vi "Main.vi"() -> ()   [LabVIEW 2018] (continued)
            n1262 = call <vilib>:"Boolean Crossing PtByPt.vi"("direction"=enum16{"either", "false-true", "true-false"}."false-true", "input"=w6697) -> ("crossing"=w6701:bool)  [unwired: 1 in]
            n1263 = call <vilib>:"Boolean Crossing PtByPt.vi"("direction"=enum16{"either", "false-true", "true-false"}."true-false", "input"=w6697) -> ("crossing"=w6702:bool)  [unwired: 1 in]
            n1264 = call "已用时间6"("Reset"=w6695) -> ("Time has Elapsed"=w6696:bool)  [unwired: 11 in, 7 out]
            n1265 = Insert Into Array(array=bool[] [] ("数组"), index=0 ("索引"), new element #1=w6701, new element #2=w6702) -> (w6705:bool[])
            n1266 = Boolean Array To Number(Boolean array=w6705) -> (number=w6706:u32)
            n1267 = case shown="0, 默认" w6706 {
              tunnel: [cluster{"Data":string[], "State":T1} {"Data"=[], "State"=enum."读扫码请求2"} ("元素") w6725 w6729] -> w6698
              tunnel: w6690 -> [_ w6726 w6730]
              frame 0, Default {
              }
              frame 1 {
                w6725 = cluster{"Data":string[], "State":T1} {"Data"=[], "State"=enum."读数据"} ("元素")
                n1268 = Enqueue Element(queue=w6726, element=w6725, timeout in ms (-1)=10 ("超时毫秒(-1)")) -> ()  [unwired: 1 in, 3 out]
              }
              frame 2 {
                w6729 = cluster{"Data":string[], "State":T1} {"Data"=["999"], "State"=enum."数据保存回复"} ("元素")
                n1269 = Enqueue Element(queue=w6730, element=w6729, timeout in ms (-1)=10 ("超时毫秒(-1)")) -> ()  [unwired: 1 in, 3 out]
              }
            }
            n1270 = case shown="真" w6696 {
              tunnel: w6690 -> [_ w6722]
              frame False {
              }
              frame True {
                n1271 = Enqueue Element(queue=w6722, element=cluster{"Data":string[], "State":T1} {"Data"=["999"], "State"=enum."数据保存回复"} ("元素"), timeout in ms (-1)=10 ("超时毫秒(-1)")) -> ()  [unwired: 1 in, 3 out]
              }
            }
          }
          frame "读数据" {
            w6756 = u16 1 items=["byte", "word", "Dword"] ("数据类型")
            w6760 = u8 132 items=["I/O (P)"=128, "Input (I)"=129, "Output (Q)"=130, "Bit Memory (M)"=131, "Data (DB)"=132, "Instance Data (DI)"=133, "Local Data (L)"=134, "Predecessor Local Data (VL)"=135] ("寄存器类型")
            n1272 = call "S7_Read.vi"("TCP"=w6734, "DB #"=u16 20, "读取长度"=u16 1, "寄存器类型"=w6760, "起始地址"=u32 6, "数据类型"=w6756) -> ("TCP"=w6755:refnum<k5>, "数据"=w6752:u32[], "error out"=w6745:errorcluster)  [unwired: 6 in, 1 out]
            n1273 = local read "ST202 Dowel Pin M0104893"() -> (w6731:string)
            n1274 = Index Array(array=w6752) -> (element=w6751:u32)  [unwired: 1 in]
            n1275 = local read "ST202 Camring 5026187"() -> (w6732:string)
            n1276 = local read "ST202 Rotor 5025805"() -> (w6733:string)
            n1277 = Equal?(x=w6751, y=u32 1) -> (x = y?=w6749:bool)
            n1278 = case shown="假" w6749 {
              tunnel: ["NG" "OK"] -> w6737
              frame False {
              }
              frame True {
              }
            }
            n1279 = Format Date/Time String(time format string (%c)="%Y-%m-%d" ("时间格式字符串(%c)")) -> (date/time string=w6739:string)  [unwired: 2 in]
            n1280 = Get Date/Time String() -> (time string=w6738:string)  [unwired: 3 in, 1 out]
            n1281 = Insert Into Array(array=string[] [] ("数组"), index=0 ("索引"), new element #1="202" ("新元素/子数组"), new element #2=w6737, new element #3=w6739, new element #4=w6738, new element #5=w6737, new element #6=w6733, new element #7=w6732, new element #8=w6731) -> (w6747:string[])
            n1282 = Enqueue Element(queue=w6746, element=w6747, error in (no error)=w6745) -> (error out=w6744:errorcluster)  [unwired: 1 in, 2 out]
            n1283 = property on="ST201数据读取(事件)" class="Bool (严格)"(error in=w6744, "Val(Sgnl)"=TRUE ("值(信号)")) -> (error out=w6735:errorcluster)  [unwired: 1 in, 1 out]
          }
          frame "数据保存回复" {
            w6776 = u8 132 items=["I/O (P)"=128, "Input (I)"=129, "Output (Q)"=130, "Bit Memory (M)"=131, "Data (DB)"=132, "Instance Data (DI)"=133, "Local Data (L)"=134, "Predecessor Local Data (VL)"=135] ("寄存器类型")
            w6777 = u16 1 items=["byte", "word", "Dword"] ("数据类型")
            n1284 = Index Array(array=w6766, index=0 ("索引")) -> (element=w6764:string)
            "数据保存请求回复201" <- w6764
            n1285 = Decimal String To Number(string=w6764, default (0L)=u32 0 ("默认(0 I32)")) -> (number=w6772:u32)  [unwired: 1 in, 1 out]
            n1286 = call "S7_Write.vi"("TCP"=w6771, "寄存器类型"=w6776, "DB #"=u16 20, "写入地址"=u32 4, "数据类型"=w6777, "写入数据"=w6772) -> ("TCP"=w6769:refnum<k5>, "error out"=w6770:errorcluster)  [unwired: 7 in, 1 out]
            n1287 = Bundle By Name(cluster=w6765, "数据保存超时1"=w6764) -> (w6763:T11)
          }
          frame "-----------------" {
          }
          frame "读扫码请求2" {
            w6792 = u8 132 items=["I/O (P)"=128, "Input (I)"=129, "Output (Q)"=130, "Bit Memory (M)"=131, "Data (DB)"=132, "Instance Data (DI)"=133, "Local Data (L)"=134, "Predecessor Local Data (VL)"=135] ("寄存器类型")
            w6793 = u16 1 items=["byte", "word", "Dword"] ("数据类型")
            w6804 = u16 0 items=["byte", "word", "Dword"] ("数据类型")
            w6806 = u8 132 items=["I/O (P)"=128, "Input (I)"=129, "Output (Q)"=130, "Bit Memory (M)"=131, "Data (DB)"=132, "Instance Data (DI)"=133, "Local Data (L)"=134, "Predecessor Local Data (VL)"=135] ("寄存器类型")
            n1288 = Unbundle By Name(w6787) -> ("看门狗"=w6795:string)
            n1289 = Decimal String To Number(string=w6795) -> (number=w6796:i32)  [unwired: 2 in, 1 out]
            n1290 = Equal?(x=w6796, y=0) -> (x = y?=w6798:bool)
            n1291 = case shown="假" w6798 {
              tunnel: [0 ("y") 1 ("y")] -> w6789
              frame False {
              }
              frame True {
              }
            }
            n1292 = local write "20"(w6789) -> ()
            n1293 = call "S7_Write.vi"("TCP"=w6788, "寄存器类型"=w6792, "DB #"=u16 20, "写入地址"=u32 22, "数据类型"=w6793, "写入数据"=w6789) -> ("TCP"=w6785:refnum<k5>, "error out"=w6784:errorcluster)  [unwired: 7 in, 1 out]
            n1294 = Number To Decimal String(number=w6789) -> (decimal integer string=w6790:string)  [unwired: 1 in]
            n1295 = Bundle By Name(cluster=w6787, "看门狗"=w6790) -> (w6786:T11)
            n1296 = call "S7_Read.vi"("TCP"=w6785, "DB #"=u16 20, "读取长度"=u16 1, "寄存器类型"=w6806, "起始地址"=u32 0, "数据类型"=w6804, "error in"=w6784) -> ("TCP"=w6803:refnum<k5>, "数据"=w6829:u32[], "读取成功"=w6816:bool, "error out"=w6800:errorcluster)  [unwired: 5 in]
            n1297 = Not(x=w6816) -> (.not. x?=w6817:bool)
            n1298 = Index Array(array=w6829, index=0 ("索引")) -> (element=w6828:u32)
            n1299 = local write "ST20通讯状态"(w6817) -> ()
            n1300 = Number To Boolean Array(number=w6828) -> (Boolean array=w6827:bool[])
            n1301 = Unbundle By Name(w6786) -> ("扫码超时2"=w6818:string)
            n1302 = Index Array(array=w6827, index=2 ("索引")) -> (element=w6822:bool)
            "ST203扫码请求" <- w6822
            n1303 = Not Equal?(x=w6818, y="999") -> (x != y?=w6819:bool)
            n1304 = Not(x=w6819) -> (.not. x?=w6820:bool)
            n1305 = call <vilib>:"Boolean Crossing PtByPt.vi"("direction"=enum16{"either", "false-true", "true-false"}."false-true", "input"=w6822) -> ("crossing"=w6826:bool)  [unwired: 1 in]
            n1306 = call <vilib>:"Boolean Crossing PtByPt.vi"("direction"=enum16{"either", "false-true", "true-false"}."true-false", "input"=w6822) -> ("crossing"=w6825:bool)  [unwired: 1 in]
            n1307 = call "已用时间21"("Reset"=w6820) -> ("Time has Elapsed"=w6821:bool)  [unwired: 11 in, 7 out]
            n1308 = Insert Into Array(array=bool[] [] ("数组"), index=0 ("索引"), new element #1=w6826, new element #2=w6825) -> (w6824:bool[])
            n1309 = Boolean Array To Number(Boolean array=w6824) -> (number=w6823:u32)
            n1310 = case shown="0, 默认" w6823 {
              tunnel: [cluster{"Data":string[], "State":T1} {"Data"=[], "State"=enum."读数据保存请求2"} ("元素") w6837 w6839] -> w6802
              tunnel: w6799 -> [_ w6838 w6840]
              frame 0, Default {
              }
              frame 1 {
                w6837 = cluster{"Data":string[], "State":T1} {"Data"=[], "State"=enum."读二维码2"} ("元素")
                n1311 = Enqueue Element(queue=w6838, element=w6837, timeout in ms (-1)=10 ("超时毫秒(-1)")) -> ()  [unwired: 1 in, 3 out]
              }
              frame 2 {
                w6839 = cluster{"Data":string[], "State":T1} {"Data"=["999"], "State"=enum."扫码回复2"} ("元素")
                n1312 = Enqueue Element(queue=w6840, element=w6839, timeout in ms (-1)=10 ("超时毫秒(-1)")) -> ()  [unwired: 1 in, 3 out]
              }
            }
            n1313 = case shown="真" w6821 {
              tunnel: w6799 -> [_ w6833]
              frame False {
              }
              frame True {
                n1314 = Enqueue Element(queue=w6833, element=cluster{"Data":string[], "State":T1} {"Data"=["999"], "State"=enum."扫码回复2"} ("元素"), timeout in ms (-1)=10 ("超时毫秒(-1)")) -> ()  [unwired: 1 in, 3 out]
              }
            }
          }
          frame "读二维码2" {
            w6853 = u16 0 items=["byte", "word", "Dword"] ("数据类型")
            w6855 = u8 132 items=["I/O (P)"=128, "Input (I)"=129, "Output (Q)"=130, "Bit Memory (M)"=131, "Data (DB)"=132, "Instance Data (DI)"=133, "Local Data (L)"=134, "Predecessor Local Data (VL)"=135] ("寄存器类型")
            n1315 = call "S7_Read.vi"("TCP"=w6852, "DB #"=u16 20, "读取长度"=u16 17, "寄存器类型"=w6855, "起始地址"=u32 42, "数据类型"=w6853) -> ("TCP"=w6850:refnum<k5>, "数据"=w6858:u32[], "error out"=w6860:errorcluster)  [unwired: 6 in, 1 out]
            n1316 = To Unsigned Word Integer(number=w6858) -> (unsigned 16bit integer=w6859:u16[])
            n1317 = call "还原为字符串.vi"("error in (no error)"=w6860, "输入数组"=w6859) -> ("error out"=w6844:errorcluster, "字符串"=w6845:string)  [unwired: 8 in]
            n1318 = Match Pattern(string=w6845, regular expression=" " ("正则表达式")) -> (before substring=w6842:string)  [unwired: 1 in, 3 out]
            n1319 = flat-sequence {
              tunnel: w6844 -> [w6862]
              tunnel: [w6862] -> w6843
              tunnel: w6842 -> [w6861]
              tunnel: [w6864] -> w6849
              tunnel: w6843 -> [w6863]
              frame #0 {
                "202二维码" <- w6861
              }
              frame #1 {
                n1320 = property on="ST203扫码请求（事件）" class="Bool (严格)"(error in=w6863, "Val(Sgnl)"=TRUE ("值(信号)")) -> (error out=w6864:errorcluster)  [unwired: 1 in, 1 out]
              }
            }
          }
          frame "扫码回复2" {
            n1321 = Array Size(array=w6872) -> (size(s)=w6875:i32)
            n1322 = case shown="3, 默认" w6875 {
              tunnel: w6872 -> [w6877 w6911]
              tunnel: w6873 -> [w6878 w6898]
              tunnel: [w6880 w6889] -> w6870
              tunnel: [w6879 w6888] -> w6869
              tunnel: [w6876 w6887] -> w6874
              frame 1 {
                w6883 = u8 132 items=["I/O (P)"=128, "Input (I)"=129, "Output (Q)"=130, "Bit Memory (M)"=131, "Data (DB)"=132, "Instance Data (DI)"=133, "Local Data (L)"=134, "Predecessor Local Data (VL)"=135] ("寄存器类型")
                w6882 = u16 1 items=["byte", "word", "Dword"] ("数据类型")
                n1323 = Index Array(array=w6877) -> (element=w6876:string)  [unwired: 1 in]
                n1324 = Decimal String To Number(string=w6876, default (0L)=u32 0 ("默认(0 I32)")) -> (number=w6886:u32)  [unwired: 1 in, 1 out]
                n1325 = call "S7_Write.vi"("TCP"=w6878, "寄存器类型"=w6883, "DB #"=u16 20, "写入地址"=u32 14, "数据类型"=w6882, "写入数据"=w6886) -> ("TCP"=w6880:refnum<k5>, "error out"=w6879:errorcluster)  [unwired: 7 in, 1 out]
              }
              frame 3, Default {
                w6901 = u8 132 items=["I/O (P)"=128, "Input (I)"=129, "Output (Q)"=130, "Bit Memory (M)"=131, "Data (DB)"=132, "Instance Data (DI)"=133, "Local Data (L)"=134, "Predecessor Local Data (VL)"=135] ("寄存器类型")
                w6900 = u16 1 items=["byte", "word", "Dword"] ("数据类型")
                w6908 = u8 132 items=["I/O (P)"=128, "Input (I)"=129, "Output (Q)"=130, "Bit Memory (M)"=131, "Data (DB)"=132, "Instance Data (DI)"=133, "Local Data (L)"=134, "Predecessor Local Data (VL)"=135] ("寄存器类型")
                w6909 = u16 1 items=["byte", "word", "Dword"] ("数据类型")
                w6915 = u8 132 items=["I/O (P)"=128, "Input (I)"=129, "Output (Q)"=130, "Bit Memory (M)"=131, "Data (DB)"=132, "Instance Data (DI)"=133, "Local Data (L)"=134, "Predecessor Local Data (VL)"=135] ("寄存器类型")
                w6914 = u16 1 items=["byte", "word", "Dword"] ("数据类型")
                n1326 = Index Array(array=w6911) -> (element #1=w6887:string, element #2=w6894:string, element #3=w6893:string)  [unwired: 3 in]
                n1327 = Equal?(x=w6893, y="OK") -> (x = y?=w6891:bool)
                n1328 = Decimal String To Number(string=w6894, default (0L)=u32 0 ("默认(0 I32)")) -> (number=w6895:u32)  [unwired: 1 in, 1 out]
                n1329 = case shown="假" w6891 {
                  tunnel: [u32 2 ("写入数据") u32 1 ("写入数据")] -> w6890
                  frame False {
                  }
                  frame True {
                  }
                }
                n1330 = call "S7_Write.vi"("TCP"=w6898, "寄存器类型"=w6915, "DB #"=u16 20, "写入地址"=u32 18, "数据类型"=w6914, "写入数据"=w6895) -> ("TCP"=w6905:refnum<k5>, "error out"=w6906:errorcluster)  [unwired: 7 in, 1 out]
                n1331 = call "S7_Write.vi"("TCP"=w6905, "寄存器类型"=w6908, "DB #"=u16 20, "写入地址"=u32 20, "数据类型"=w6909, "写入数据"=w6890, "error in"=w6906) -> ("TCP"=w6897:refnum<k5>, "error out"=w6896:errorcluster)  [unwired: 6 in, 1 out]
                n1332 = Decimal String To Number(string=w6887, default (0L)=u32 0 ("默认(0 I32)")) -> (number=w6904:u32)  [unwired: 1 in, 1 out]
                n1333 = call "S7_Write.vi"("TCP"=w6897, "寄存器类型"=w6901, "DB #"=u16 20, "写入地址"=u32 14, "数据类型"=w6900, "写入数据"=w6904, "error in"=w6896) -> ("TCP"=w6889:refnum<k5>, "error out"=w6888:errorcluster)  [unwired: 6 in, 1 out]
              }
            }
            "扫码请求回复202" <- w6874
            n1334 = Bundle By Name(cluster=w6868, "扫码超时2"=w6874) -> (w6867:T11)
          }
          frame "-- --------------" {
          }
          frame "读数据保存请求2" {
            w6931 = u16 0 items=["byte", "word", "Dword"] ("数据类型")
            w6933 = u8 132 items=["I/O (P)"=128, "Input (I)"=129, "Output (Q)"=130, "Bit Memory (M)"=131, "Data (DB)"=132, "Instance Data (DI)"=133, "Local Data (L)"=134, "Predecessor Local Data (VL)"=135] ("寄存器类型")
            n1335 = call "S7_Read.vi"("TCP"=w6929, "DB #"=u16 20, "读取长度"=u16 1, "寄存器类型"=w6933, "起始地址"=u32 0, "数据类型"=w6931) -> ("TCP"=w6927:refnum<k5>, "数据"=w6954:u32[], "error out"=w6925:errorcluster)  [unwired: 6 in, 1 out]
            n1336 = Index Array(array=w6954, index=0 ("索引")) -> (element=w6953:u32)
            n1337 = Number To Boolean Array(number=w6953) -> (Boolean array=w6952:bool[])
            n1338 = Unbundle By Name(w6930) -> ("数据保存超时2"=w6943:string)
            n1339 = Index Array(array=w6952, index=3 ("索引")) -> (element=w6947:bool)
            "ST202数据读取" <- w6947
            n1340 = Not Equal?(x=w6943, y="999") -> (x != y?=w6944:bool)
            n1341 = Not(x=w6944) -> (.not. x?=w6945:bool)
            n1342 = call <vilib>:"Boolean Crossing PtByPt.vi"("direction"=enum16{"either", "false-true", "true-false"}."false-true", "input"=w6947) -> ("crossing"=w6948:bool)  [unwired: 1 in]
            n1343 = call <vilib>:"Boolean Crossing PtByPt.vi"("direction"=enum16{"either", "false-true", "true-false"}."true-false", "input"=w6947) -> ("crossing"=w6949:bool)  [unwired: 1 in]
            n1344 = call "已用时间22"("Reset"=w6945) -> ("Time has Elapsed"=w6946:bool)  [unwired: 11 in, 7 out]
            n1345 = Insert Into Array(array=bool[] [] ("数组"), index=0 ("索引"), new element #1=w6948, new element #2=w6949) -> (w6950:bool[])
            n1346 = Boolean Array To Number(Boolean array=w6950) -> (number=w6951:u32)
            n1347 = case shown="1" w6951 {
              tunnel: [cluster{"Data":string[], "State":T1} {"Data"=[], "State"=enum."看门狗"} ("元素") w6959 w6963] -> w6924
              tunnel: w6928 -> [_ w6960 w6964]
              frame 0, Default {
              }
              frame 1 {
                w6959 = cluster{"Data":string[], "State":T1} {"Data"=[], "State"=enum."读数据2"} ("元素")
                n1348 = Enqueue Element(queue=w6960, element=w6959, timeout in ms (-1)=10 ("超时毫秒(-1)")) -> ()  [unwired: 1 in, 3 out]
              }
              frame 2 {
                w6963 = cluster{"Data":string[], "State":T1} {"Data"=["999"], "State"=enum."数据保存回复2"} ("元素")
                n1349 = Enqueue Element(queue=w6964, element=w6963, timeout in ms (-1)=10 ("超时毫秒(-1)")) -> ()  [unwired: 1 in, 3 out]
              }
            }
            n1350 = case shown="真" w6946 {
              tunnel: w6928 -> [_ w6956]
              frame False {
              }
              frame True {
                n1351 = Enqueue Element(queue=w6956, element=cluster{"Data":string[], "State":T1} {"Data"=["999"], "State"=enum."数据保存回复2"} ("元素"), timeout in ms (-1)=10 ("超时毫秒(-1)")) -> ()  [unwired: 1 in, 3 out]
              }
            }
          }
          frame "读数据2" {
            w6979 = i16 2 ("精度(6)")
            w6991 = u16 1 items=["byte", "word", "Dword"] ("数据类型")
            w6989 = u8 132 items=["I/O (P)"=128, "Input (I)"=129, "Output (Q)"=130, "Bit Memory (M)"=131, "Data (DB)"=132, "Instance Data (DI)"=133, "Local Data (L)"=134, "Predecessor Local Data (VL)"=135] ("寄存器类型")
            w6993 = u16 1 items=["byte", "word", "Dword"] ("数据类型")
            w6995 = u8 132 items=["I/O (P)"=128, "Input (I)"=129, "Output (Q)"=130, "Bit Memory (M)"=131, "Data (DB)"=132, "Instance Data (DI)"=133, "Local Data (L)"=134, "Predecessor Local Data (VL)"=135] ("寄存器类型")
            n1352 = call "S7_Read.vi"("TCP"=w6986, "DB #"=u16 20, "读取长度"=u16 4, "寄存器类型"=w6989, "起始地址"=u32 60, "数据类型"=w6991) -> ("TCP"=w6981:refnum<k5>, "数据"=w6972:u32[], "error out"=w6980:errorcluster)  [unwired: 6 in, 1 out]
            n1353 = Divide(x=w6972, y=u32[] [100, 100, 100, 100]) -> (x/y=w6974:dbl[])
            n1354 = Index Array(array=w6974) -> (element #1=w6975:dbl, element #2=w6976:dbl, element #3=w6977:dbl, element #4=w6978:dbl)  [unwired: 4 in]
            n1355 = Number To Fractional String(number=w6975, precision (6)=w6979) -> (F-format string=w6971:string)  [unwired: 2 in]
            n1356 = Number To Fractional String(number=w6976, precision (6)=w6979) -> (F-format string=w6970:string)  [unwired: 2 in]
            n1357 = Number To Fractional String(number=w6977, precision (6)=w6979) -> (F-format string=w6969:string)  [unwired: 2 in]
            n1358 = Number To Fractional String(number=w6978, precision (6)=w6979) -> (F-format string=w6968:string)  [unwired: 2 in]
            n1359 = call "S7_Read.vi"("TCP"=w6981, "DB #"=u16 20, "读取长度"=u16 1, "寄存器类型"=w6995, "起始地址"=u32 12, "数据类型"=w6993, "error in"=w6980) -> ("TCP"=w6985:refnum<k5>, "数据"=w7008:u32[], "error out"=w6967:errorcluster)  [unwired: 5 in, 1 out]
            n1360 = Index Array(array=w7008) -> (element=w7007:u32)  [unwired: 1 in]
            n1361 = Equal?(x=w7007, y=u32 1) -> (x = y?=w7006:bool)
            n1362 = case shown="假" w7006 {
              tunnel: ["NG" "OK"] -> w7003
              frame False {
              }
              frame True {
              }
            }
            n1363 = Format Date/Time String(time format string (%c)="%Y-%m-%d" ("时间格式字符串(%c)")) -> (date/time string=w7005:string)  [unwired: 2 in]
            n1364 = Get Date/Time String() -> (time string=w7004:string)  [unwired: 3 in, 1 out]
            n1365 = Insert Into Array(array=string[] [] ("数组"), index=0 ("索引"), new element #1="203" ("新元素/子数组"), new element #2=w7003, new element #3=w7005, new element #4=w7004, new element #5=w7003, new element #6=w6971, new element #7=w6970, new element #8=w6969, new element #9=w6968) -> (w6965:string[])
            n1366 = flat-sequence {
              tunnel: w6967 -> [w7010]
              tunnel: [w7010] -> w6966
              tunnel: w6965 -> [w7009]
              tunnel: [w7012] -> w6983
              tunnel: w6966 -> [w7011]
              frame #0 {
                "202读取数据" <- w7009
              }
              frame #1 {
                n1367 = property on="ST203数据读取（事件）" class="Bool (严格)"(error in=w7011, "Val(Sgnl)"=TRUE ("值(信号)")) -> (error out=w7012:errorcluster)  [unwired: 1 in, 1 out]
              }
            }
          }
          frame "数据保存回复2" {
            w7027 = u8 132 items=["I/O (P)"=128, "Input (I)"=129, "Output (Q)"=130, "Bit Memory (M)"=131, "Data (DB)"=132, "Instance Data (DI)"=133, "Local Data (L)"=134, "Predecessor Local Data (VL)"=135] ("寄存器类型")
            w7024 = u16 1 items=["byte", "word", "Dword"] ("数据类型")
            n1368 = Index Array(array=w7018, index=0 ("索引")) -> (element=w7030:string)
            "数据保存请求回复202" <- w7030
            n1369 = Decimal String To Number(string=w7030, default (0L)=u32 0 ("默认(0 I32)")) -> (number=w7031:u32)  [unwired: 1 in, 1 out]
            n1370 = call "S7_Write.vi"("TCP"=w7023, "寄存器类型"=w7027, "DB #"=u16 20, "写入地址"=u32 16, "数据类型"=w7024, "写入数据"=w7031) -> ("TCP"=w7020:refnum<k5>, "error out"=w7019:errorcluster)  [unwired: 7 in, 1 out]
            n1371 = Bundle By Name(cluster=w7022, "数据保存超时2"=w7030) -> (w7021:T11)
          }
          frame "------------" {
          }
          frame "错误" {
            n1372 = Flush Queue(queue=w7039) -> ()  [unwired: 1 in, 3 out]
            n1373 = Flush Queue(queue=w7038) -> ()  [unwired: 1 in, 3 out]
            n1374 = call "S7_Close.vi"("TCP Connection Ref"=w7042) -> ("error out"=w7040:errorcluster)  [unwired: 10 in]
            n1375 = call <vilib>:"Clear Errors.vi"("error in (no error)"=w7040) -> ()  [unwired: 5 in, 2 out]
          }
          frame "退出" {
            n1376 = Release Queue(queue=w7051) -> ()  [unwired: 2 in, 3 out]
            n1377 = Release Queue(queue=w7050) -> ()  [unwired: 2 in, 3 out]
            n1378 = call "S7_Close.vi"("TCP Connection Ref"=w7049) -> ("error out"=w7047:errorcluster)  [unwired: 10 in]
          }
          frame "看门狗" {
            w7064 = "\r" ("正则表达式")
            w7082 = u16 0 items=["byte", "word", "Dword"] ("数据类型")
            w7080 = u8 132 items=["I/O (P)"=128, "Input (I)"=129, "Output (Q)"=130, "Bit Memory (M)"=131, "Data (DB)"=132, "Instance Data (DI)"=133, "Local Data (L)"=134, "Predecessor Local Data (VL)"=135] ("寄存器类型")
            w7092 = u8 132 items=["I/O (P)"=128, "Input (I)"=129, "Output (Q)"=130, "Bit Memory (M)"=131, "Data (DB)"=132, "Instance Data (DI)"=133, "Local Data (L)"=134, "Predecessor Local Data (VL)"=135] ("寄存器类型")
            w7093 = u16 1 items=["byte", "word", "Dword"] ("数据类型")
            n1379 = Unbundle By Name(w7085) -> ("看门狗"=w7095:string)
            n1380 = Decimal String To Number(string=w7095) -> (number=w7096:i32)  [unwired: 2 in, 1 out]
            n1381 = Equal?(x=w7096, y=0) -> (x = y?=w7098:bool)
            n1382 = case shown="假" w7098 {
              tunnel: [0 ("y") 1 ("y")] -> w7086
              frame False {
              }
              frame True {
              }
            }
            "20" <- w7086
            n1383 = call "S7_Write.vi"("TCP"=w7090, "寄存器类型"=w7092, "DB #"=u16 20, "写入地址"=u32 22, "数据类型"=w7093, "写入数据"=w7086) -> ("TCP"=w7072:refnum<k5>, "error out"=w7071:errorcluster)  [unwired: 7 in, 1 out]
            n1384 = Number To Decimal String(number=w7086) -> (decimal integer string=w7087:string)  [unwired: 1 in]
            n1385 = Bundle By Name(cluster=w7085, "看门狗"=w7087) -> (w7084:T11)
            n1386 = call "S7_Read.vi"("TCP"=w7072, "DB #"=u16 20, "读取长度"=u16 120, "寄存器类型"=w7080, "起始地址"=u32 70, "数据类型"=w7082, "error in"=w7071) -> ("TCP"=w7057:refnum<k5>, "数据"=w7074:u32[], "error out"=w7056:errorcluster)  [unwired: 5 in, 1 out]
            n1387 = To Unsigned Word Integer(number=w7074) -> (unsigned 16bit integer=w7073:u16[])
            n1388 = call "还原为字符串.vi"("输入数组"=w7073) -> ("字符串"=w7075:string)  [unwired: 9 in, 1 out]
            n1389 = for {
              N: 6 -> [_]
              tunnel: w7075 -> [w7115]
              tunnel: [w7114] -> w7083 mode=indexing
              shift-right: [w7110] -> _
              shift-left: 0 ("长度（剩余）") -> [w7112]
              n1390 = String Subset(string=w7115, offset (0)=w7112, length (rest)=20 ("长度（剩余）")) -> (substring=w7114:string)
              n1391 = Add(x=w7112, y=20) -> (x+y=w7110:i32)
            }
            n1392 = Index Array(array=w7083) -> (element #1=w7070:string, element #2=w7069:string, element #3=w7068:string, element #4=w7067:string, element #5=w7066:string, element #6=w7065:string)  [unwired: 6 in]
            n1393 = Match Pattern(string=w7070, regular expression=w7064) -> (before substring=→"ST202 Rotor 5025805":string)  [unwired: 1 in, 3 out]
            n1394 = Match Pattern(string=w7069, regular expression=w7064) -> (before substring=→"ST202 Camring 5026187":string)  [unwired: 1 in, 3 out]
            n1395 = Match Pattern(string=w7068, regular expression=w7064) -> (before substring=→"ST202 Dowel Pin M0104893":string)  [unwired: 1 in, 3 out]
            n1396 = Match Pattern(string=w7067, regular expression=w7064) -> (before substring=→"ST301 Vane 5004737":string)  [unwired: 1 in, 3 out]
            n1397 = Match Pattern(string=w7066, regular expression=w7064) -> (before substring=→"ST301 Dowel Pin 5024533":string)  [unwired: 1 in, 3 out]
            n1398 = Match Pattern(string=w7065, regular expression=w7064) -> (before substring=→"ST301 Dowel Pin 5020282":string)  [unwired: 1 in, 3 out]
            n1399 = disable-structure shown="启用" {
              disable-tunnel: w7057 -> [w7099 w7103]
              disable-tunnel: [w7099 w7106] -> w7054
              disable-tunnel: w7056 -> [w7100 w7104]
              disable-tunnel: [w7100 w7105] -> w7055
              frame Disabled {
              }
              frame Enabled {
                w7108 = u8 132 items=["I/O (P)"=128, "Input (I)"=129, "Output (Q)"=130, "Bit Memory (M)"=131, "Data (DB)"=132, "Instance Data (DI)"=133, "Local Data (L)"=134, "Predecessor Local Data (VL)"=135] ("寄存器类型")
                w7102 = u16 1 items=["byte", "word", "Dword"] ("数据类型")
                n1400 = local read "80产品型号"() -> (w7101:u32)
                n1401 = call "S7_Write.vi"("TCP"=w7103, "寄存器类型"=w7108, "DB #"=u16 20, "写入地址"=u32 190, "数据类型"=w7102, "写入数据"=w7101, "error in"=w7104) -> ("TCP"=w7106:refnum<k5>, "error out"=w7105:errorcluster)  [unwired: 6 in, 1 out]
              }
            }
          }
        }
      }
      n1402 = while {
        tunnel: w107 -> [w613]
        tunnel: w144 -> [w612]
        stop <- w611 stop-if-true
        n1403 = event shown="[0] 超时" {
          selector: _ -> [_ _ _ _ _ _ _ _ _ _ _ _]
          dyn-events: _ -> [_ _ _ _ _ _ _ _ _ _ _ _]
          timeout: 10 -> [_ _ _ _ _ _ _ _ _ _ _ _]
          tunnel: w613 -> [_ w621 _ _ _ _ _ _ _ _ _ _]
          tunnel: w612 -> [_ w620 _ _ _ _ _ _ _ _ _ _]
          tunnel: [FALSE w617 FALSE FALSE FALSE FALSE FALSE FALSE FALSE FALSE FALSE FALSE] -> w611
          event Timeout {
            n1404 = event-data() -> ()  [unwired: 1 in, 3 out]
          }
          event Panel Close {
            n1405 = event-data() -> ()  [unwired: 1 in, 3 out]
            n1406 = call <vilib>:"DB Tools Close Connection.vi"("error in (no error)"=w621, "connection reference"=w620) -> ()  [unwired: 5 in, 1 out]
            n1407 = Two Button Dialog(message="确定退出？" ("消息")) -> (T button?=w618:bool)  [unwired: 2 in]
            n1408 = case shown="真" w618 {
              tunnel: [FALSE TRUE] -> w617
              frame False {
              }
              frame True {
                n1409 = flat-sequence {
                  frame #0 {
                    n1410 = property on="错误信息" class="LstBox (严格)"() -> ("Item Names"=w626:string[])  [unwired: 2 in, 2 out]
                    n1411 = Array Size(array=w626) -> (size(s)=w625:i32)
                    n1412 = Equal To 0?(x=w625) -> (x = 0?=w624:bool)
                    n1413 = case shown="假" w624 {
                      tunnel: w626 -> [w627 _]
                      frame False {
                        n1414 = call <vilib>:"Check if File or Folder Exists.vi"("path"=path "D:/Alarm_Log") -> ("error out"=w643:errorcluster, "file or folder exists?"=w644:bool, "dup path"=w642:path)  [unwired: 8 in]
                        n1415 = case shown="真" w644 {
                          tunnel: w643 -> [w659 w660]
                          tunnel: w642 -> [w658 w661]
                          tunnel: [w657 w661] -> w641
                          tunnel: [w656 w660] -> w636
                          frame False {
                            n1416 = Create Folder(path (use dialog)=w658, error in=w659) -> (created path=w657:path, error out=w656:errorcluster)  [unwired: 1 in, 1 out]
                          }
                          frame True {
                          }
                        }
                        n1417 = Format Date/Time String(time format string (%c)="%Y%m%d" ("时间格式字符串(%c)")) -> (date/time string=w639:string)  [unwired: 2 in]
                        n1418 = Concatenate Strings(w639, ".txt" ("字符串")) -> (w637:string)
                        n1419 = Build Path(base path=w641, name or relative path=w637) -> (appended path=w630:path)
                        n1420 = call <vilib>:"Check if File or Folder Exists.vi"("error in (no error)"=w636, "path"=w630) -> ("error out"=w634:errorcluster, "file or folder exists?"=w635:bool, "dup path"=w633:path)  [unwired: 7 in]
                        n1421 = case shown="假" w635 {
                          tunnel: w634 -> [_ w649]
                          tunnel: w633 -> [_ w648]
                          tunnel: [string[] [] ("array of strings") w647] -> w631
                          frame False {
                          }
                          frame True {
                            n1422 = Read from Text File(file (use dialog)=w648, error in=w649) -> (text=w650:string)  [unwired: 2 in, 3 out]
                            n1423 = Search and Replace String(replace all?=TRUE ("替换全部？(F)"), input string=w650, search string="\n" ("搜索字符串"), replace string="\\" ("替换字符串(\"\")")) -> (result string=w654:string)  [unwired: 4 in, 3 out]
                            n1424 = String To Path(string=w654) -> (path=w655:path)
                            n1425 = Path to Array of Strings(0:w655) -> (2:w647:string[])  [unwired: 1 out]
                          }
                        }
                        n1426 = Array Size(array=w627) -> (size(s)=w632:i32)
                        n1427 = Insert Into Array(array=w627, index=w632, new element=w631) -> (w629:string[])
                        n1428 = Write to Text File(file (use dialog)=w630, text=w629) -> (error out=w628:errorcluster)  [unwired: 2 in, 2 out]
                        n1429 = call <vilib>:"Clear Errors.vi"("error in (no error)"=w628) -> ()  [unwired: 5 in, 2 out]
                      }
                      frame True {
                      }
                    }
                  }
                  frame #1 {
                    n1430 = control-ref of="本VI"() -> (w662:refnum<vi>)
                    n1431 = property class="VI"(reference=w662, "FP.State"=T6."Closed" ("前面板窗口:状态")) -> ()  [unwired: 1 in, 2 out]
                  }
                }
              }
            }
            n1432 = local write "退出"(w617) -> ()
          }
          event "返回": Value Change {
            n1433 = event-data() -> ()  [unwired: 1 in, 3 out]
            n1434 = local write "Main Tab"(T2."Running" ("Main Tab")) -> ()
          }
          event "登录界面": Value Change {
            w666 = "" ("输入管理员密码")
            n1435 = event-data() -> ()  [unwired: 1 in, 3 out]
            n1436 = local write "输入管理员密码"(w666) -> ()
            n1437 = local write "登录状态"(w666) -> ()
            n1438 = local write "Main Tab"(T2."Setting" ("Main Tab")) -> ()
          }
          event "登录": Value Change {
            n1439 = event-data() -> ()  [unwired: 1 in, 3 out]
            n1440 = local read "Code"() -> (w675:string)
            n1441 = Equal?(x="输入管理员密码", y="15505240996") -> (x = y?=w669:bool)
            n1442 = Equal?(x="输入管理员密码", y=w675) -> (x = y?=w674:bool)
            n1443 = case shown="真" w669 {
              frame False {
              }
              frame True {
                "Main Tab" <- T2."Monitor" ("Main Tab")
              }
            }
            n1444 = case shown="真" w674 {
              tunnel: ["登录失败！" ("登录状态") "登录成功！" ("登录状态")] -> w673
              frame False {
              }
              frame True {
                w679 = TRUE ("可见")
                n1445 = property on="Rework界面" class="Bool"("Visible"=w679) -> ()  [unwired: 2 in, 2 out]
                n1446 = property on="修改密码" class="Bool"("Visible"=w679) -> ()  [unwired: 2 in, 2 out]
                n1447 = property on="注销" class="Bool"("Visible"=w679) -> ()  [unwired: 2 in, 2 out]
                n1448 = local write "Main Tab"(T2."Running" ("Main Tab")) -> ()
              }
            }
            "登录状态" <- w673
          }
          event "修改密码界面返回", "登录界面返回", "Rework返回": Value Change {
            n1449 = event-data() -> ()  [unwired: 1 in, 3 out]
            n1450 = local write "Main Tab"(T2."Running" ("Main Tab")) -> ()
          }
          event "Rework界面": Value Change {
            w683 = FALSE ("503")
            w686 = "" ("输入需要Rework的一维码：")
            n1451 = event-data() -> ()  [unwired: 1 in, 3 out]
            n1452 = local write "80"(w683) -> ()
            n1453 = local write "101"(w683) -> ()
            n1454 = local write "102"(w683) -> ()
            n1455 = local write "202"(w683) -> ()
            n1456 = local write "203"(w683) -> ()
            n1457 = local write "301"(w683) -> ()
            n1458 = local write "302"(w683) -> ()
            n1459 = local write "401"(w683) -> ()
            n1460 = local write "403"(w683) -> ()
            n1461 = local write "502"(w683) -> ()
            n1462 = local write "503"(w683) -> ()
            n1463 = local write "601"(w683) -> ()
            n1464 = local write "602"(w683) -> ()
            n1465 = local write "70"(w683) -> ()
            n1466 = local write "Rework状态"(w686) -> ()
            n1467 = local write "输入需要Rework的一维码："(w686) -> ()
            n1468 = local write "Main Tab"(T2."Rework" ("Main Tab")) -> ()
          }
          event "102", "202", "301", "401", "502", "503", "601", "70", "101", "203", "302", "403", "602": Value Change {
            w687 = cluster{u32, u32}[] [{1985280, 1985280}, {6618880, 6618880}, {1985280, 1985280}, {6618880, 6618880}] ("颜色[4]")
            n1469 = event-data() -> ()  [unwired: 1 in, 3 out]
            n1470 = property on="101" class="Bool (严格)"("Colors [4]"=w687) -> ()  [unwired: 2 in, 2 out]
            n1471 = property on="102" class="Bool (严格)"("Colors [4]"=w687) -> ()  [unwired: 2 in, 2 out]
            n1472 = property on="202" class="Bool (严格)"("Colors [4]"=w687) -> ()  [unwired: 2 in, 2 out]
            n1473 = property on="203" class="Bool (严格)"("Colors [4]"=w687) -> ()  [unwired: 2 in, 2 out]
            n1474 = property on="301" class="Bool (严格)"("Colors [4]"=w687) -> ()  [unwired: 2 in, 2 out]
            n1475 = property on="302" class="Bool (严格)"("Colors [4]"=w687) -> ()  [unwired: 2 in, 2 out]
            n1476 = property on="401" class="Bool (严格)"("Colors [4]"=w687) -> ()  [unwired: 2 in, 2 out]
            n1477 = property on="403" class="Bool (严格)"("Colors [4]"=w687) -> ()  [unwired: 2 in, 2 out]
            n1478 = property on="502" class="Bool (严格)"("Colors [4]"=w687) -> ()  [unwired: 2 in, 2 out]
            n1479 = property on="503" class="Bool (严格)"("Colors [4]"=w687) -> ()  [unwired: 2 in, 2 out]
            n1480 = property on="601" class="Bool (严格)"("Colors [4]"=w687) -> ()  [unwired: 2 in, 2 out]
            n1481 = property on="602" class="Bool (严格)"("Colors [4]"=w687) -> ()  [unwired: 2 in, 2 out]
            n1482 = property on="70" class="Bool (严格)"("Colors [4]"=w687) -> ()  [unwired: 2 in, 2 out]
          }
          event "注销": Value Change {
            w689 = FALSE ("可见")
            n1483 = event-data() -> ()  [unwired: 1 in, 3 out]
            n1484 = property on="Rework界面" class="Bool"("Visible"=w689) -> ()  [unwired: 2 in, 2 out]
            n1485 = property on="修改密码" class="Bool"("Visible"=w689) -> ()  [unwired: 2 in, 2 out]
            n1486 = property on="注销" class="Bool"("Visible"=w689) -> ()  [unwired: 2 in, 2 out]
          }
          event "修改密码": Value Change {
            w691 = "" ("修改密码状态")
            n1487 = event-data() -> ()  [unwired: 1 in, 3 out]
            n1488 = local write "Main Tab"(T2."Modify" ("Main Tab")) -> ()
            n1489 = local write "修改密码状态"(w691) -> ()
            n1490 = local write "新密码"(w691) -> ()
            n1491 = local write "初始密码"(w691) -> ()
          }
          event "确认修改密码": Value Change {
            n1492 = event-data() -> ()  [unwired: 1 in, 3 out]
            n1493 = local read "Code"() -> (w696:string)
            n1494 = Equal?(x="初始密码", y=w696) -> (x = y?=w695:bool)
            n1495 = case shown="真" w695 {
              tunnel: ["初始密码错误" ("修改密码状态") w701] -> w694
              frame False {
              }
              frame True {
                w703 = "Code" ("subkeyName")
                n1496 = call "Write Registry.vi"("value"=w703, "data"="新密码", "subkeyName"=w703) -> ("error out"=w702:errorcluster)  [unwired: 8 in]
                n1497 = case shown="无错误" w702 {
                  tunnel: ["修改密码成功" ("修改密码状态") "修改密码失败" ("修改密码状态")] -> w701
                  tunnel: "新密码" -> [w704 _]
                  frame No Error {
                    n1498 = local write "Code"(w704) -> ()
                  }
                  frame Error {
                  }
                }
              }
            }
            "修改密码状态" <- w694
          }
          event "OP70画曲线": Value Change {
            # "注：分支0：未收到请求，查找下一个PLC请求\n      分支1：扫码请求，读取码\n      分支2：扫码复位，回复给PLC的也要复位"
            n1499 = event-data() -> ()  [unwired: 1 in, 3 out]
            n1500 = call "检查曲线文件.vi"("Folder Path"=path "D:/op70" ("路径")) -> ("Error Out"=w709:errorcluster, "Exit?"=w711:bool, "曲线文件路径"=w710:path)  [unwired: 7 in, 1 out]
            n1501 = case shown="真" w711 {
              tunnel: w710 -> [_ w726]
              tunnel: w709 -> [w722 w725]
              tunnel: [w722 w724] -> w708
              frame False {
              }
              frame True {
                n1502 = flat-sequence {
                  tunnel: [w730] -> w727
                  tunnel: w726 -> [w729]
                  tunnel: w725 -> [w731]
                  tunnel: [w729] -> w723
                  tunnel: w727 -> [w744]
                  tunnel: [w749] -> w724
                  tunnel: w723 -> [w747]
                  frame #0 {
                    n1503 = call "EXCEL 画曲线.vi"("错误输入（无错误）"=w731, "路径"=w729) -> ("error IO"=w730:errorcluster, "XY图"=→"XY图":cluster{"X":dbl, "Y":dbl}[])  [unwired: 8 in]
                    "曲线文件路径" <- w729
                  }
                  frame #1 {
                    n1504 = local read "70二维码"() -> (w735:string)
                    n1505 = Format Date/Time String(time format string (%c)="%Y%m%d" ("时间格式字符串(%c)")) -> (date/time string=w732:string)  [unwired: 2 in]
                    n1506 = call "图片保存(subaru).vi"("一维码"=w732) -> ("dup path"=w737:path)  [unwired: 9 in, 1 out]
                    n1507 = Build Path(base path=w737, name or relative path=w735) -> (appended path=w750:path)
                    n1508 = call <vilib>:"Check if File or Folder Exists.vi"("path"=w750) -> ("error out"=w751:errorcluster, "file or folder exists?"=w752:bool)  [unwired: 8 in, 1 out]
                    n1509 = Concatenate Strings(w735, "ST70.BMP" ("字符串")) -> (w753:string)
                    n1510 = case shown="假" w752 {
                      tunnel: w750 -> [w757 w759]
                      tunnel: [w756 w759] -> w736
                      tunnel: w751 -> [w755 w758]
                      tunnel: [w754 w758] -> _
                      frame False {
                        n1511 = Create Folder(path (use dialog)=w757, error in=w755) -> (created path=w756:path, error out=w754:errorcluster)  [unwired: 1 in, 1 out]
                      }
                      frame True {
                      }
                    }
                    n1512 = Build Path(base path=w736, name or relative path=w753) -> (appended path=w746:path)
                    n1513 = call "文件路径.vi"("文件路径"=w746, "文件格式"=".BMP") -> ("新路径"=w740:path)  [unwired: 9 in]
                    n1514 = invoke on="XY图" class="XYGraph (严格)" method="Export Image"(error in=w744, "FileType"=enum32{"BMP", "EPS", "EMF", "PICT"}."BMP" ("文件类型"), "Target"=enum32{"File", "Clipboard"}."File" ("目标"), "Path"=w740, "HideGrid"=FALSE ("隐藏网格"), "Overwrite"=TRUE ("隐藏网格")) -> (error out=w743:errorcluster)  [unwired: 2 in, 7 out]
                    n1515 = Move(source path=w747, error in=w743, 9:TRUE ("覆盖(F)"), 10:w736) -> (error out=w749:errorcluster)  [unwired: 1 in, 2 out]
                    "error IO" <- w744
                  }
                }
              }
            }
            n1516 = case shown="错误" w708 {
              frame No Error {
              }
              frame Error {
                n1517 = property on="错误信息" class="LstBox (严格)"() -> ("Item Names"=w718:string[])  [unwired: 2 in, 2 out]
                n1518 = Format Date/Time String(time format string (%c)="%Y-%m-%d %H:%M:%S" ("时间格式字符串(%c)")) -> (date/time string=w720:string)  [unwired: 2 in]
                n1519 = Concatenate Strings(w720, "  " ("字符串"), "ST70 画曲线错误") -> (w716:string)
                n1520 = Insert Into Array(array=w718, index=0 ("索引"), new element=w716) -> (w715:string[])
                n1521 = property on="错误信息" class="LstBox (严格)"("Item Names"=w715) -> ()  [unwired: 2 in, 2 out]
              }
            }
            "OP70画曲线" <- FALSE ("ST10画曲线")
          }
        }
        n1522 = Wait (ms)(milliseconds to wait=u32 10 ("等待时间（毫秒）")) -> ()  [unwired: 1 out]
      }
      n1523 = while {
        tunnel: w144 -> [w763]
        tunnel: w107 -> [w762]
        tunnel: w147 -> [w779]
        tunnel: w145 -> [w780]
        tunnel: w141 -> [w777]
        tunnel: w140 -> [w778]
        tunnel: w125 -> [w775]
        tunnel: w123 -> [w776]
        tunnel: w120 -> [w773]
        tunnel: w118 -> [w774]
        tunnel: w137 -> [w771]
        tunnel: w136 -> [w772]
        tunnel: w115 -> [w769]
        tunnel: w114 -> [w770]
        tunnel: w116 -> [w760]
        tunnel: w111 -> [w766]
        tunnel: w110 -> [w765]
        tunnel: w109 -> [w761]
        stop <- w781 stop-if-true
        n1524 = event shown="[1] \"ST101扫码请求（事件）\": 值改变" {
          selector: _ -> [_ _ _ _ _ _ _ _ _ _ _ _ _ _ _ _ _ _ _ _ _ _ _ _ _ _ _ _ _ _]
          dyn-events: _ -> [_ _ _ _ _ _ _ _ _ _ _ _ _ _ _ _ _ _ _ _ _ _ _ _ _ _ _ _ _ _]
          timeout: 10 -> [_ _ _ _ _ _ _ _ _ _ _ _ _ _ _ _ _ _ _ _ _ _ _ _ _ _ _ _ _ _]
          tunnel: w763 -> [_ w976 w1043 w1178 w1196 w1300 w1343 w1452 w1495 w1601 w1642 w1752 w1795 w1898 w1940 w2052 w2095 w2201 w2242 w2349 w2395 w2501 w2544 w2651 w2696 w2802 w2856 w2980 w3083 w3214]
          tunnel: w762 -> [_ w975 w1032 w1177 w1195 w1301 w1342 w1451 w1494 w1600 w1643 w1751 w1794 w1897 w1939 w2051 w2094 w2200 w2243 w2348 w2394 w2500 w2545 w2652 w2695 w2801 w2855 w2975 w3082 w3213]
          tunnel: w780 -> [_ _ w1069 _ _ _ _ _ _ _ _ _ _ _ _ _ _ _ _ _ _ _ _ _ _ _ _ _ _ _]
          tunnel: w779 -> [_ w1003 w1068 w1163 w1194 _ _ _ _ _ _ _ _ _ _ _ _ _ _ _ _ _ _ _ _ _ _ _ _ _]
          tunnel: w778 -> [_ _ _ _ _ _ w1369 _ _ _ _ _ _ _ _ _ _ _ _ _ _ _ _ _ _ _ _ _ _ _]
          tunnel: w777 -> [_ _ _ _ _ w1299 w1368 w1450 w1493 _ _ _ _ _ _ _ _ _ _ _ _ _ _ _ _ _ _ _ _ _]
          tunnel: w776 -> [_ _ _ _ _ _ _ _ _ _ w1668 _ _ _ _ _ _ _ _ _ _ _ _ _ _ _ _ _ _ _]
          tunnel: w775 -> [_ _ _ _ _ _ _ _ _ w1599 w1667 w1750 w1793 _ _ _ _ _ _ _ _ _ _ _ _ _ _ _ _ _]
          tunnel: w774 -> [_ _ _ _ _ _ _ _ _ _ _ _ _ _ w1968 _ _ _ _ _ _ _ _ _ _ _ _ _ _ _]
          tunnel: w773 -> [_ _ _ _ _ _ _ _ _ _ _ _ _ w1902 w1967 w2050 w2093 _ _ _ _ _ _ _ _ _ _ _ _ _]
          tunnel: w772 -> [_ _ _ _ _ _ _ _ _ _ _ _ _ _ _ _ _ _ w2260 _ _ _ _ _ _ _ _ _ _ _]
          tunnel: w771 -> [_ _ _ _ _ _ _ _ _ _ _ _ _ _ _ _ _ w2199 w2259 w2353 w2413 _ _ _ _ _ _ _ _ _]
          tunnel: w770 -> [_ _ _ _ _ _ _ _ _ _ _ _ _ _ _ _ _ _ _ _ _ _ w2540 _ _ _ _ _ _ _]
          tunnel: w769 -> [_ _ _ _ _ _ _ _ _ _ _ _ _ _ _ _ _ _ _ _ _ w2499 w2560 w2647 w2689 _ _ _ _ _]
          tunnel: [errorcluster {"status"=FALSE, "code"=0, "source"=""} ("error out") w985 w1033 w1150 w1191 w1297 w1341 w1449 w1490 w1598 w1639 w1749 w1792 w1901 w1942 w2049 w2090 w2198 w2239 w2352 w2398 w2498 w2543 w2650 w2694 w2800 w2841 w2986 w3081 w3212] -> w767
          tunnel: ["" "ST101 扫码请求错误" "ST101 数据读取错误" "ST102 扫码请求错误" "ST102 数据保存错误" "ST202 扫码请求错误" "ST202 数据读取错误" "ST203 扫码请求错误" "ST203 数据读取错误" "ST301 扫码请求错误" "ST301 数据读取错误" "ST302 扫码请求错误" "ST302 数据读取错误" "ST401 扫码请求错误" "ST401 数据读取错误" "ST403 扫码请求错误" "ST403 数据读取错误" "ST502 扫码请求错误" "ST502 数据读取错误" "ST503 扫码请求错误" "ST503 数据读取错误" "ST601 扫码请求错误" "ST601 数据读取错误" "ST602 扫码请求错误" "ST602 数据读取错误" "ST802 扫码请求错误" w2840 w2983 "查询数据库失败" "Rework失败"] -> w768
          tunnel: w766 -> [_ _ _ _ _ _ _ _ _ _ _ _ _ _ _ _ _ _ _ _ _ _ _ _ _ w2797 w2853 w2987 _ _]
          tunnel: w765 -> [_ _ _ _ _ _ _ _ _ _ _ _ _ _ _ _ _ _ _ _ _ _ _ _ _ _ _ _ _ _]
          event Timeout {
            n1525 = event-data() -> ()  [unwired: 1 in, 3 out]
          }
          event "ST101扫码请求（事件）": Value Change {
            w971 = "ORDER BY ID DESC" ("查询语句")
            # "判断数据库中有无该条码,目前只查询最后插入的1w条数据"
            n1526 = event-data() -> ()  [unwired: 1 in, 1 out]
            n1527 = local read "101 二维码"() -> (w964:string)
            n1528 = call "Albert_SQL_101.vi"("表名"="Online", "error in (no error)"=w975, "查询语句"=w971, "connection reference"=w976) -> ("error out"=w972:errorcluster, "数据"=w969:string[][], "connection reference out"=w973:T12)  [unwired: 5 in]
            n1529 = call "Albert_SQL_101.vi"("表名"="Offline", "error in (no error)"=w972, "查询语句"=w971, "connection reference"=w973) -> ("error out"=w966:errorcluster, "数据"=w965:string[][], "connection reference out"=w967:T12)  [unwired: 5 in]
            n1530 = call "Albert_Arr_QueryString.vi"("字符串"=w964, "2D Arr Input"=w965) -> ("2D Arr Output"=w963:string[][])  [unwired: 9 in]
            n1531 = call "Albert_Arr_QueryString.vi"("字符串"=w964, "2D Arr Input"=w969) -> ("2D Arr Output"=w968:string[][])  [unwired: 9 in]
            n1532 = Format Date/Time String(time format string (%c)="%Y-%m-%d" ("时间格式字符串(%c)")) -> (date/time string=w994:string)  [unwired: 2 in]
            n1533 = Get Date/Time String() -> (time string=w993:string)  [unwired: 3 in, 1 out]
            n1534 = Insert Into Array(array=string[] [] ("数组"), index=0 ("索引"), new element #1=w994, new element #2=w993, new element #3=w964) -> (w990:string[])
            n1535 = Insert Into Array(array=string[][] [] ("数组"), index (row)=0 ("索引 (行)"), new element=w990) -> (w987:string[][])  [unwired: 1 in]
            n1536 = Matrix Size(0:w963) -> (1:w982:i32)  [unwired: 1 out]
            n1537 = Matrix Size(0:w968) -> (1:w1005:i32)  [unwired: 1 out]
            n1538 = Transpose 2D Array(2D array=w987) -> (transposed array=w986:string[][])
            n1539 = Equal?(x=w982, y=0) -> (x = y?=w979:bool)
            n1540 = Equal?(x=w1005, y=0) -> (x = y?=w981:bool)
            n1541 = property on="ST10-1_DATA" class="MCListbox (严格)"("ItemNames"=w986) -> ()  [unwired: 2 in, 2 out]
            n1542 = And(x=w979, y=w981) -> (x .and. y?=w980:bool)
            n1543 = case shown="假" w980 {
              tunnel: w967 -> [_ _]
              tunnel: w966 -> [w1012 w1029]
              tunnel: ["2" ("左扫码请求回复") w1028] -> w996
              tunnel: [w1012 w1029] -> w985
              tunnel: w979 -> [w1011 _]
              tunnel: w963 -> [w1010 _]
              tunnel: [w1009 "100"] -> w978
              tunnel: [w1008 "OK"] -> w977
              tunnel: w968 -> [w1007 _]
              frame False {
                n1544 = case shown="假" w1011 {
                  tunnel: w1010 -> [w1019 _]
                  tunnel: [w1015 w1021] -> w1009
                  tunnel: [w1014 w1020] -> w1008
                  tunnel: w1007 -> [_ w1022]
                  frame False {
                    w1017 = 0 ("索引 (行)")
                    n1545 = Index Array(array=w1019, index (row) #1=w1017, index (col) #1=0 ("禁用的索引 (列)"), index (row) #2=w1017, index (col) #2=1 ("禁用的索引 (列)")) -> (element #1=w1015:string, element #2=w1014:string)
                  }
                  frame True {
                    w1025 = 0 ("索引 (行)")
                    n1546 = Index Array(array=w1022, index (row) #1=w1025, index (col) #1=0 ("禁用的索引 (列)"), index (row) #2=w1025, index (col) #2=1 ("禁用的索引 (列)")) -> (element #1=w1021:string, element #2=w1020:string)
                  }
                }
              }
              frame True {
                n1547 = case shown="无错误" w1029 {
                  tunnel: ["1" ("左扫码请求回复") "3" ("左扫码请求回复")] -> w1028
                  frame No Error {
                  }
                  frame Error {
                  }
                }
              }
            }
            "101 上一站号" <- w978
            "101 上一站结果" <- w977
            n1548 = Insert Into Array(array=string[] [] ("数组"), index=0 ("索引"), new element #1=w996, new element #2=w978, new element #3=w977) -> (w999:string[])
            n1549 = Bundle By Name(cluster=cluster{"Data":string[], "State":T1} {"Data"=[], "State"=enum."PLC通讯初始化"} ("元素"), "Data"=w999, "State"=状态2."扫码回复") -> (w998:cluster{"Data":string[], "State":T1})
            n1550 = Enqueue Element(queue=w1003, element=w998) -> ()  [unwired: 2 in, 3 out]
            "ST101扫码请求（事件）" <- FALSE ("ST10左扫码请求")
          }
          event "ST101数据读取（事件）": Value Change {
            w1040 = 0 ("索引 (行)")
            n1551 = event-data() -> ()  [unwired: 1 in, 1 out]
            n1552 = local read "101 二维码"() -> (w1034:string)
            n1553 = Dequeue Element(queue=w1069, timeout in ms (-1)=10 ("超时毫秒(-1)")) -> (element=w1054:string[])  [unwired: 1 in, 3 out]
            n1554 = Concatenate Strings("Where QRCode='" ("查询语句"), w1034, "'" ("字符串")) -> (w1042:string)
            n1555 = call "SQL_Select.vi"("要读取的列名"=string[] ["Rework_Status"], "表名"="Online", "error in (no error)"=w1032, "查询语句"=w1042, "查询条件"=TRUE, "connection reference"=w1043) -> ("error out"=w1035:errorcluster, "数据"=w1041:string[][], "connection reference out"=w1036:T12)  [unwired: 3 in]
            n1556 = Index Array(array=w1041, index (row)=w1040, index (col)=w1040) -> (element=w1039:string)
            n1557 = Equal?(x=w1039, y="T") -> (x = y?=w1037:bool)
            n1558 = case shown="假" w1037 {
              tunnel: [w1088 w1092] -> w1060
              tunnel: w1054 -> [w1078 w1095]
              tunnel: [w1079 w1091] -> w1033
              tunnel: w1034 -> [w1076 w1094]
              tunnel: w1042 -> [_ w1093]
              tunnel: w1036 -> [w1082 w1106]
              tunnel: w1035 -> [w1081 w1105]
              frame False {
                n1559 = Format Date/Time String(time format string (%c)="%Y-%m-%d_%H:%M" ("时间格式字符串(%c)")) -> (date/time string=w1074:string)  [unwired: 2 in]
                n1560 = local read "产品型号"() -> (w1072:string)
                n1561 = Insert Into Array(array=w1078, index=2 ("索引"), new element #1=w1074, new element #2=w1076) -> (w1073:string[])
                n1562 = Insert Into Array(array=w1073, new element=w1072) -> (w1071:string[])  [unwired: 1 in]
                n1563 = call "SQL_Insert.vi"("表名"="Online", "error in (no error)"=w1081, "值"=w1071, "列名"=string[] ["Last_Station", "Last_Result", "Online_Time", "QRCode", "ST101_Date", "ST101_Time", "ST101_Package_Result", "ST101_Shaft_M0102049", "ST101_Form_Seal_5026859", "ST101_Dowel_Pin_5024532", "ST101_Dowel_Pin_5020281", "ST101_Control_Plat_5025303", "ST101_Flange_M0104918", "ST101_Camera_Shield", "ST101_Seal_Ring_Below_TestValue", "ST101_Seal_Ring_Below_SetValue", "ST101_Seal_Ring_Above_TestValue", "ST101_Seal_Ring_Above_SetValue", "ProductType"], "connection reference"=w1082) -> ("error out"=w1079:errorcluster)  [unwired: 5 in, 1 out]
                n1564 = Unbundle By Name(w1079) -> ("status"=w1087:bool)
                n1565 = Equal?(x=w1076, y="") -> (x = y?=w1085:bool)
                n1566 = Or(x=w1087, y=w1085) -> (x .or. y?=w1084:bool)
                n1567 = case shown="真" w1084 {
                  tunnel: ["1" ("数据保存请求回复") "2" ("数据保存请求回复")] -> w1088
                  frame False {
                  }
                  frame True {
                  }
                }
              }
              frame True {
                w1101 = 0 ("索引 (行)")
                n1568 = call "SQL_Select.vi"("要读取的列名"=string[] ["[101]"], "表名"="Rework_List", "error in (no error)"=w1105, "查询语句"=w1093, "查询条件"=TRUE, "connection reference"=w1106) -> ("error out"=w1096:errorcluster, "数据"=w1102:string[][], "connection reference out"=w1097:T12)  [unwired: 3 in]
                n1569 = Index Array(array=w1102, index (row)=w1101, index (col)=w1101) -> (element=w1100:string)
                n1570 = Equal?(x=w1100, y="T") -> (x = y?=w1098:bool)
                n1571 = case shown="真" w1098 {
                  tunnel: w1097 -> [w1114 w1133]
                  tunnel: w1096 -> [w1115 w1132]
                  tunnel: w1095 -> [w1113 w1139]
                  tunnel: w1094 -> [w1110 w1134]
                  tunnel: w1093 -> [w1112 w1126]
                  tunnel: [w1109 w1125] -> w1092
                  tunnel: [w1111 w1124] -> w1091
                  frame False {
                    n1572 = call "SQL_Update.vi"("查询语句"=w1112, "表名"="Online", "error in (no error)"=w1115, "列名对应的值"=w1113, "列名"=string[] ["Last_Station", "Last_Result", "ST101_Date", "ST101_Time", "ST101_Package_Result", "ST101_Shaft_M0102049", "ST101_Form_Seal_5026859", "ST101_Dowel_Pin_5024532", "ST101_Dowel_Pin_5020281", "ST101_Control_Plat_5025303", "ST101_Flange_M0104918", "ST101_Camera_Shield", "ST101_Seal_Ring_Below_TestValue", "ST101_Seal_Ring_Below_SetValue", "ST101_Seal_Ring_Above_TestValue", "ST101_Seal_Ring_Above_SetValue"], "connection reference"=w1114) -> ("error out"=w1111:errorcluster)  [unwired: 4 in, 1 out]
                    n1573 = Unbundle By Name(w1111) -> ("status"=w1119:bool)
                    n1574 = Equal?(x=w1110, y="") -> (x = y?=w1117:bool)
                    n1575 = Or(x=w1119, y=w1117) -> (x .or. y?=w1116:bool)
                    n1576 = case shown="假" w1116 {
                      tunnel: ["1" ("数据保存请求回复") "2" ("数据保存请求回复")] -> w1109
                      frame False {
                      }
                      frame True {
                      }
                    }
                  }
                  frame True {
                    n1577 = Delete From Array(array=w1139, length=2 ("长度"), index=0 ("索引")) -> (deleted portion=w1127:string[], array with subset deleted=w1136:string[])
                    n1578 = call "SQL_Update.vi"("查询语句"=w1126, "表名"="Online", "error in (no error)"=w1132, "列名对应的值"=w1127, "列名"=string[] ["Last_Station", "Last_Result"], "connection reference"=w1133) -> ("error out"=w1131:errorcluster, "connection reference 2"=w1130:T12)  [unwired: 4 in]
                    n1579 = call "SQL_Update.vi"("查询语句"=w1126, "表名"="Rework", "error in (no error)"=w1131, "列名对应的值"=w1136, "列名"=string[] ["ST101_Date", "ST101_Time", "ST101_Package_Result", "ST101_Shaft_M0102049", "ST101_Form_Seal_5026859", "ST101_Dowel_Pin_5024532", "ST101_Dowel_Pin_5020281", "ST101_Control_Plat_5025303", "ST101_Flange_M0104918", "ST101_Camera_Shield", "ST101_Seal_Ring_Below_TestValue", "ST101_Seal_Ring_Below_SetValue", "ST101_Seal_Ring_Above_TestValue", "ST101_Seal_Ring_Above_SetValue"], "connection reference"=w1130) -> ("error out"=w1124:errorcluster)  [unwired: 4 in, 1 out]
                    n1580 = Unbundle By Name(w1124) -> ("status"=w1142:bool)
                    n1581 = Equal?(x="", y=w1134) -> (x = y?=w1141:bool)
                    n1582 = Or(x=w1142, y=w1141) -> (x .or. y?=w1140:bool)
                    n1583 = case shown="假" w1140 {
                      tunnel: ["1" ("数据保存请求回复") "2" ("数据保存请求回复")] -> w1125
                      frame False {
                      }
                      frame True {
                      }
                    }
                  }
                }
              }
            }
            n1584 = Insert Into Array(array=string[] [] ("数组"), index=0 ("索引"), new element=w1060) -> (w1066:string[])
            n1585 = Delete From Array(array=w1054, length=2 ("长度"), index=0 ("索引")) -> (array with subset deleted=w1051:string[])  [unwired: 1 out]
            n1586 = Bundle By Name(cluster=cluster{"Data":string[], "State":T1} {"Data"=[], "State"=enum."PLC通讯初始化"} ("元素"), "Data"=w1066, "State"=状态2."数据保存回复") -> (w1059:cluster{"Data":string[], "State":T1})
            n1587 = Insert Into Array(array=w1051, index=2 ("索引"), new element=w1034) -> (w1049:string[])
            n1588 = Enqueue Element(queue=w1068, element=w1059) -> ()  [unwired: 2 in, 3 out]
            n1589 = Insert Into Array(array=string[][] [] ("数组"), index (row)=0 ("索引 (行)"), new element=w1049) -> (w1056:string[][])  [unwired: 1 in]
            n1590 = Transpose 2D Array(2D array=w1056) -> (transposed array=w1055:string[][])
            n1591 = property on="ST10-1_DATA" class="MCListbox (严格)"("ItemNames"=w1055) -> ()  [unwired: 2 in, 2 out]
            "ST101数据读取（事件）" <- FALSE ("ST10数据读取（事件）")
          }
          event "ST102扫码请求（事件）": Value Change {
            n1592 = event-data() -> ()  [unwired: 1 in, 1 out]
            n1593 = local write "ST102扫码请求（事件）"(FALSE ("ST102扫码请求（事件）")) -> ()
            n1594 = local read "102 二维码"() -> (w1146:string)
